vi "stopServos.vi"() -> (0 "error out":errorcluster)   [LabVIEW 2011]
uses:
  GlobalSerial.vi
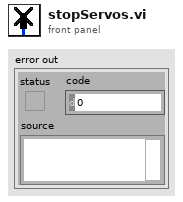
[diagram p1: front panel]
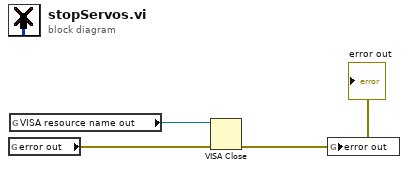
[diagram p0: block diagram]
diagram:
  n1 = global read "GlobalSerial.vi" "error out"() -> (w3:errorcluster)
  n2 = global read "GlobalSerial.vi" "VISA resource name out"() -> (w2:refnum<visa-resource-name>)
  n3 = VISA Close(VISA resource name=w2, error in (no error)=w3) -> (error out=w1:errorcluster)
  "error out" <- w1
  n4 = global write "GlobalSerial.vi" "error out"(w1) -> ()
